vi "practica22.vi"() -> ()   [LabVIEW 2013]
panel:
  out "NS  2":bool
  in  "stop":bool
  in  "D":bool
  in  "C 4":bool
  in  "B":bool
  in  "A":bool
  out "NS":bool
  out "EO 2":bool
  out "EO":bool
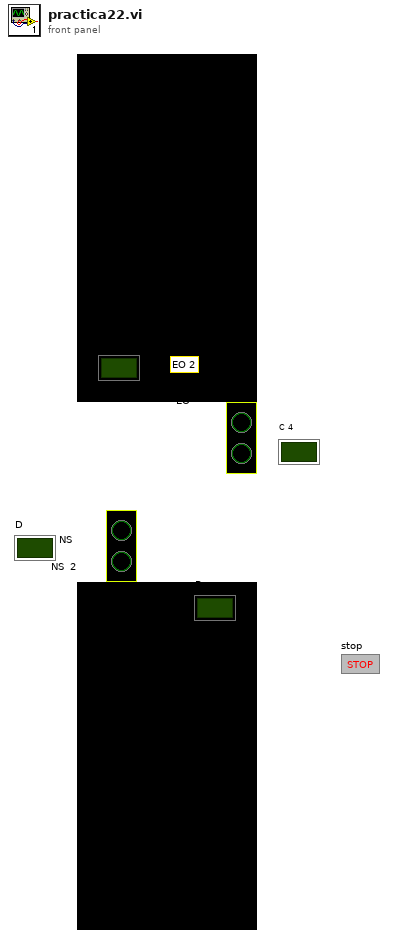
[diagram p1: front panel]
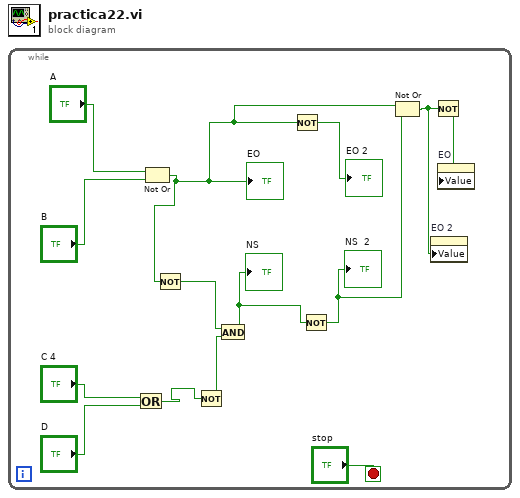
[diagram p0: block diagram]
diagram:
  n1 = while {
    stop <- "stop" stop-if-true
    n2 = Or(x="C 4", y="D") -> (x .or. y?=w9:bool)
    n3 = Not Or(1:"B", 2:"A") -> (0:w3:bool)
    "EO" <- w3
    n4 = Not(x=w3) -> (.not. x?=w8:bool)
    n5 = Not(x=w9) -> (.not. x?=w7:bool)
    n6 = And(x=w8, y=w7) -> (x .and. y?=w6:bool)
    "NS" <- w6
    n7 = Not(x=w3) -> (.not. x?=→"EO 2":bool)
    n8 = Not(x=w6) -> (.not. x?=w4:bool)
    "NS  2" <- w4
    n9 = Not Or(1:w4, 2:w3) -> (0:w1:bool)
    n10 = property on="EO 2" class="Bool (strict)"("Value"=w1) -> ()  [unwired: 2 in, 2 out]
    n11 = Not(x=w1) -> (.not. x?=w2:bool)
    n12 = property on="EO" class="Bool (strict)"("Value"=w2) -> ()  [unwired: 2 in, 2 out]
  }
